vi "Get Target IP Address.vi"(8 "error in (no error)":errorcluster, 11 "Node Ptr":T1 format="%.0x") -> (0 "error out":errorcluster, 1 "found":bool, 2 "target address":string, 3 "Item Ref out":T1 format="%.0x")   [LabVIEW 2017, in "DSF System Explorer.lvlib"]
uses:
  DSF System Explorer.lvlib
  <vilib>/NI Veristand/Custom Device API/Custom Device Item Ref.ctl
  NationalInstruments.VeriStand.SystemDefinitionAPI
  <vilib>/NI Veristand/Custom Device API/Custom Device API.lvlib
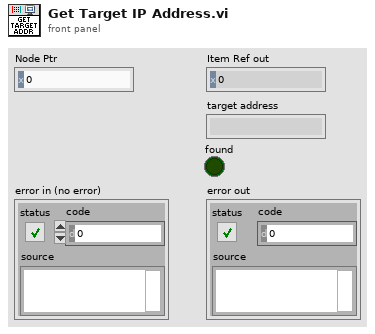
[diagram p1: front panel]
types:
  T1 = typedef "Custom Device API.lvlib/Custom Device Item Ref.ctl" = u64
  T2 = typedef "Custom Device API.lvlib/Custom Device Pointer.ctl" = refnum<k24>
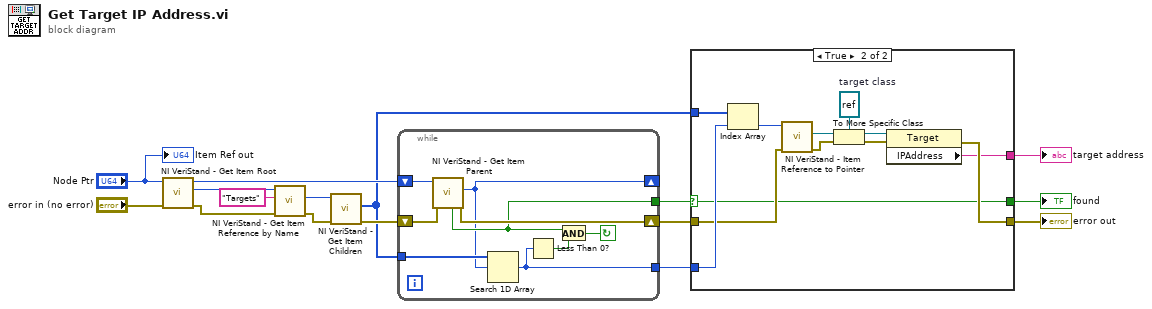
[diagram p0: block diagram]
diagram:
  n1 = call <vilib>:"NI VeriStand - Get Item Root.vi"("error in (no error)"="error in (no error)", "Item Ref in"="Node Ptr") -> ("error out"=w12:errorcluster, "Root Ref out"=w16:T1, "Item Ref out"=w9:T1)  [unwired: 6 in, 1 out]
  n2 = call <vilib>:"NI VeriStand - Get Item Reference by Name.vi"("error in (no error)"=w12, "Item Name"="Targets", "Parent Ref in"=w16) -> ("error out"=w11:errorcluster, "Item Ref"=w14:T1)  [unwired: 5 in, 2 out]
  n3 = call <vilib>:"NI VeriStand - Get Item Children.vi"("error in (no error)"=w11, "Item Ref in"=w14) -> ("error out"=w10:errorcluster, "Child Refs"=w5:T1[])  [unwired: 6 in, 2 out]
  n4 = while {
    shift-right: [w18] -> _
    shift-left: w9 -> [w25]
    shift-right: [w23] -> w7
    shift-left: w10 -> [w24]
    tunnel: w5 -> [w22]
    tunnel: [w19] -> w6
    tunnel: [w17] -> w4
    stop <- w20 continue-if-true
    n5 = call <vilib>:"NI VeriStand - Get Item Parent.vi"("error in (no error)"=w24, "Item Ref in"=w25) -> ("error out"=w23:errorcluster, "Parent Ref"=w18:T1, "Found"=w19:bool)  [unwired: 6 in, 1 out]
    n6 = Search 1D Array(1D array=w22, element=w18) -> (index of element=w17:i32)  [unwired: 1 in]
    n7 = Less Than 0?(x=w17) -> (x < 0?=w21:bool)
    n8 = And(x=w19, y=w21) -> (x .and. y?=w20:bool)
  }
  n9 = case shown="True" w6 {
    selector: w6 -> [w26 w28]
    tunnel: w7 -> [w27 w33]
    tunnel: w5 -> [_ w39]
    tunnel: w4 -> [_ w38]
    tunnel: [w27 w30] -> w3
    tunnel: [w26 w28] -> w2
    tunnel: [_ w29] -> w1
    frame False {
    }
    frame True {
      w35 = refnum<k24> refnum  # target class
      n10 = Index Array(array=w39, index=w38) -> (element=w34:T1)
      n11 = call <vilib>:"NI VeriStand - Item Reference to Pointer.vi"("error in (no error)"=w33, "Item Ref in"=w34) -> ("error out"=w32:errorcluster, "Node Pointer"=w36:T2)  [unwired: 6 in, 2 out]
      n12 = To More Specific Class(target class=w35, reference=w36, error in=w32) -> (specific class reference=w37:refnum<k24>, error out=w31:errorcluster)
      n13 = property class="Target"(reference=w37, error in=w31) -> (error out=w30:errorcluster, "IPAddress"=w29:string)  [unwired: 1 out]
    }
  }
  "error out" <- w3
  "target address" <- w1
  "found" <- w2
  "Item Ref out" <- "Node Ptr"
